vi "Handle Mode.vi"(0 "reference in":refnum<class "PM_Group.lvclass">, 11 "error in (no error)":errorcluster) -> (4 "reference out":refnum<class "PM_Group.lvclass">, 15 "error out":errorcluster)   [LabVIEW 2019]
uses:
  PM_Group.lvclass
  D:/GIT H4000/H4000/src/Device_class/Device.lvclass
  D:/GIT H4000/H4000/src/Proccess_class/Proccess.lvclass
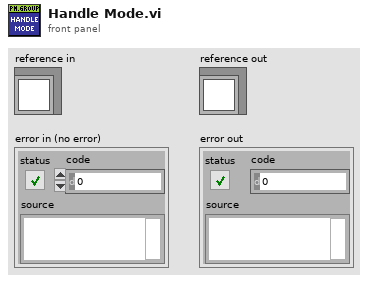
[diagram p1: front panel]
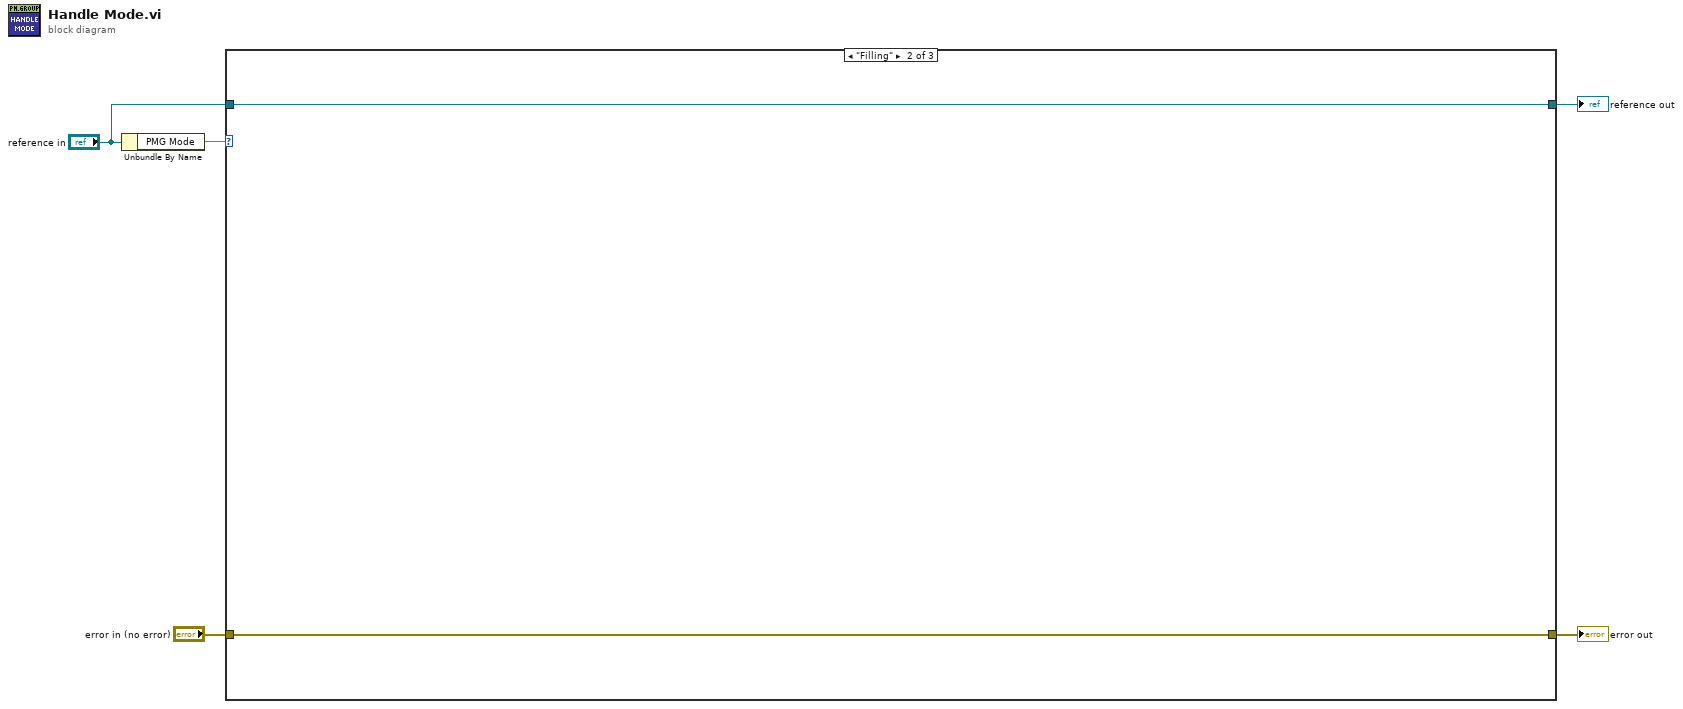
[diagram p0: block diagram]
diagram:
  n1 = Unbundle By Name("reference in") -> ("PMG Mode"=w5)
  n2 = case shown="\"Filling\"" w5 {
    tunnel: "reference in" -> [w7 w9 w11]
    tunnel: [w7 w9 w11] -> w3
    tunnel: [w6 w8 w10] -> w2
    tunnel: "error in (no error)" -> [w6 w8 w10]
    frame "Idel" {
    }
    frame "Filling" {
    }
    frame "Pressure" {
    }
  }
  "error out" <- w2
  "reference out" <- w3
